vi "Main.vi"(11 "Module Admin":refnum<class "Delacor_lib_QMH_Module Admin.lvclass">) -> ()   [LabVIEW 2020, in "Settings Editor.lvlib"]
doc: "This template is based off of the Queued Message Handler design pattern and the Queued Message Handler project template that ships with LabVIEW.\n\nThe main difference is that the queue is private to this module and communication between modules is performed via Broadcast and Request events.\n\nRequest events are wrapped in public API methods and are handled in the Event Handling Loop (EHL) of this VI. Any module can register for Broadcast events sent by this module. The EHL generates messages based on user interface actions.\n\nThe Message Handling Loop (MHL) processes messages generated by the EHL, or by other messages. The messages are string values, so new messages can be added easily to the Message Cases case structure in the MHL. Each message cluster can also provide an optional value for Message Data, which is a variant that can be converted to whatever message-specific data is required.\n_____\nBased on Delacor QMH Project Template 4.0.0.47.\n_____\nBased on DQMH Project Template 6.0.0.91."
uses:
  Settings Editor.lvlib
  DAQmx Trigger Settings--cluster.ctl
  DAQmx Timing--cluster.ctl
  DAQmx Config--cluster.ctl
  <vilib>/Delacor/Delacor QMH/Libraries/Module Admin_class/Delacor_lib_QMH_Module Admin.lvclass
  Module Data--cluster.ctl
  Settings--cluster.ctl
  Stop Argument--cluster.ctl
  <vilib>/Delacor/Delacor QMH/Libraries/Message Queue_class/Delacor_lib_QMH_Message Queue.lvclass/Delacor_lib_QMH_Message Queue.ctl
  Update Application Settings Argument--cluster.ctl
  Update Application Settings (Reply Payload)--cluster.ctl
  <vilib>/Delacor/Delacor QMH/Libraries/Module Admin_class/Delacor_lib_QMH_Module Admin.lvclass/Delacor_lib_QMH_Module Admin.ctl
  <vilib>/Delacor/Delacor QMH/Libraries/Message Queue_class/Delacor_lib_QMH_Enqueue Message (Single).vi
  <vilib>/Delacor/Delacor QMH/Libraries/Module Admin_class/Delacor_lib_QMH_Get External Launch.vi
  <vilib>/Utility/error.llb/Error Cluster From Error Code.vi
  <vilib>/ErrorRing/Error Ring.xnode
  <vilib>/Delacor/Delacor QMH/Libraries/Message Queue_class/Delacor_lib_QMH_Message Queue.lvclass
panel:
  in  "Config Something":bool
  in  "Config CAM":bool
  in  "Config DAQ":bool
  in  "DAQmx Settings":T1(tab)=enum."Timing Settings"
  in  "Hardware \nConfig Cluster":T2=[{"Physical channels"="Dev1/ai0", "Channel Name"="pd", "Unit"=0, "Min Voltage"=-1.0, "Max Voltage"=1.0}, {"Physical channels"="Dev1/ai1", "Channel Name"="pdh", "Unit"=0, "Min Voltage"=-0.5, "Max Voltage"=0.5}] {"Unit" items=["Volts", "From Custom Scale"]}
  in  "DAQmx \nTiming Settings":T3={"rate"=1000000.0, "source"="OnboardClock", "sample mode"=10178, "samples per channel"=200000} {"sample mode" items=["Finite Samples"=10178, "Continuous Samples"=10123, "Hardware Timed Single Point"=12522]; "rate" format="%0.2f"}
  in  "Trigger Settings":T4={"Trigger Type"=enum."No Trigger", "Digital Start"={"Source"="", "Digital Start Trigger Edge"=10280}, "Digital Pause"={"Source"="", "Digital Pause Trigger Pause When"=10192}, "Digital Reference"={"Source"="", "Digital Start Trigger Edge"=10280, "Digital Reference Pretrigger Samples"=0}, "Analog Start"={"Source"="", "Analog Slope"=10280, "Analog Start Trigger Hysteresis"=0.0, "Analog Start Trigger Level"=0.0}, "Analog Pause"={"Source"="", "Analog Start Trigger Level"=0.0, "Analog Pause Trigger Pause When"=10093}, "Analog Reference"={"Source"="", "Slope"=10280, "Pretrigger Samples"=0, "Level"=0.0}, "Time Start"={"Select Time\nManually"=FALSE, "When"=timestamp(0 s since 1904-01-01)}} {"Time Start"."When" format="%<%x %.3X>T"; "Analog Reference"."Level" format="%0.2f"; "Analog Reference"."Slope" items=["Rising"=10280, "Falling"=10171]; "Analog Pause"."Analog Pause Trigger Pause When" items=["Above Level"=10093, "Below Level"=10107]; "Analog Pause"."Analog Start Trigger Level" format="%0.2f"; "Analog Start"."Analog Start Trigger Level" format="%0.2f"; "Analog Start"."Analog Start Trigger Hysteresis" format="%.2f"; "Analog Start"."Analog Slope" items=["Rising"=10280, "Falling"=10171]; "Digital Reference"."Digital Start Trigger Edge" items=["Rising"=10280, "Falling"=10171]; "Digital Pause"."Digital Pause Trigger Pause When" items=["High"=10192, "Low"=10214]; "Digital Start"."Digital Start Trigger Edge" items=["Rising"=10280, "Falling"=10171]}
  in  "Calibration Array":cluster{"Slope":dbl, "Intercept":dbl}[](array[cluster])=[{"Slope"=1.0, "Intercept"=0.0}, {"Slope"=1.0, "Intercept"=0.0}]
  in  "Cancel":bool
  in  "OK":bool
  in  "Log File Base Path":path=path "C:/Logged Files/26Jan2022/test.tdms"
  out "error out":errorcluster
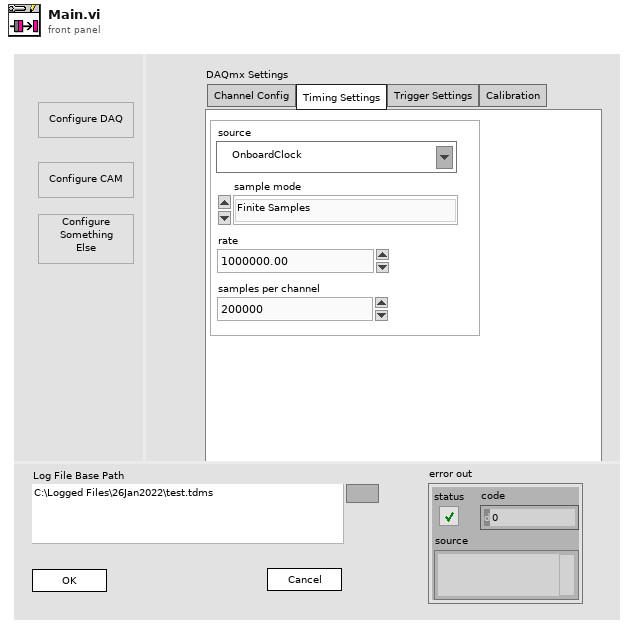
[diagram p1: front panel]
types:
  T1 = enum32{"Channel Config", "Timing Settings", "Trigger Settings", "Calibration"}
  T2 = typedef "Settings Editor.lvlib/DAQmx Config--cluster.ctl" = cluster{"Physical channels":tag, "Channel Name":string, "Unit":i32, "Min Voltage":dbl, "Max Voltage":dbl}[]
  T3 = typedef "Settings Editor.lvlib/DAQmx Timing--cluster.ctl" = cluster{"rate":dbl, "source":tag, "sample mode":i32, "samples per channel":i32}
  T4 = typedef "Settings Editor.lvlib/DAQmx Trigger Settings--cluster.ctl" = cluster{"Trigger Type":enum32{"No Trigger", "Digital Start", "Digital Pause", "Digital Reference", "Analog Start", "Analog Pause", "Analog Reference", "Time Start"}, "Digital Start":cluster{"Source":tag, "Digital Start Trigger Edge":i32}, "Digital Pause":cluster{"Source":tag, "Digital Pause Trigger Pause When":i32}, "Digital Reference":cluster{"Source":tag, "Digital Start Trigger Edge":i32, "Digital Reference Pretrigger Samples":u32}, "Analog Start":cluster{"Source":string, "Analog Slope":i32, "Analog Start Trigger Hysteresis":dbl, "Analog Start Trigger Level":dbl}, "Analog Pause":cluster{"Source":string, "Analog Start Trigger Level":dbl, "Analog Pause Trigger Pause When":i32}, "Analog Reference":cluster{"Source":string, "Slope":i32, "Pretrigger Samples":u32, "Level":dbl}, "Time Start":cluster{"Select Time\nManually":bool, "When":timestamp}}
  T5 = typedef "Settings Editor.lvlib/Request Events--cluster.ctl" = cluster{"Stop Module":refnum<user-event>, "Show Panel":refnum<user-event>, "Hide Panel":refnum<user-event>, "Get Module Execution Status":refnum<user-event>, "Show Diagram":refnum<user-event>, "Update Application Settings":refnum<user-event>}
  T6 = typedef "Settings Editor.lvlib/Module Data--cluster.ctl" = cluster{"Settings":T7}
  T7 = typedef "Settings Editor.lvlib/Settings--cluster.ctl" = cluster{"Calibration Array":cluster{"Slope":dbl, "Offset":dbl}[], "Hardware Config Cluster":T2, "Trigger Settings":T4, "Log File Base Path":path, "DAQmx Timing Settings":T3}
  T8 = enum32{"invalid lock state", "Not Locked", "Locked (No Password)", "Password-protected"}
  T9 = typedef "Settings Editor.lvlib/Stop Argument--cluster.ctl" = cluster{"Origin":string, "Exit via Stop Module Req?":bool, "Wait for Module to stop?":bool}
  T10 = typedef "Settings Editor.lvlib/Update Application Settings Argument--cluster.ctl" = cluster{"Wait Notifier":refnum<notifier>, "wait for reply":bool}
  T11 = enum32{"Invalid", "Standard", "Closed", "Hidden", "Minimized", "Maximized"}
  T12 = typedef "Settings Editor.lvlib/Update Application Settings (Reply Payload)--cluster.ctl" = cluster{"Settings":T7, "Update Settings_error":errorcluster}
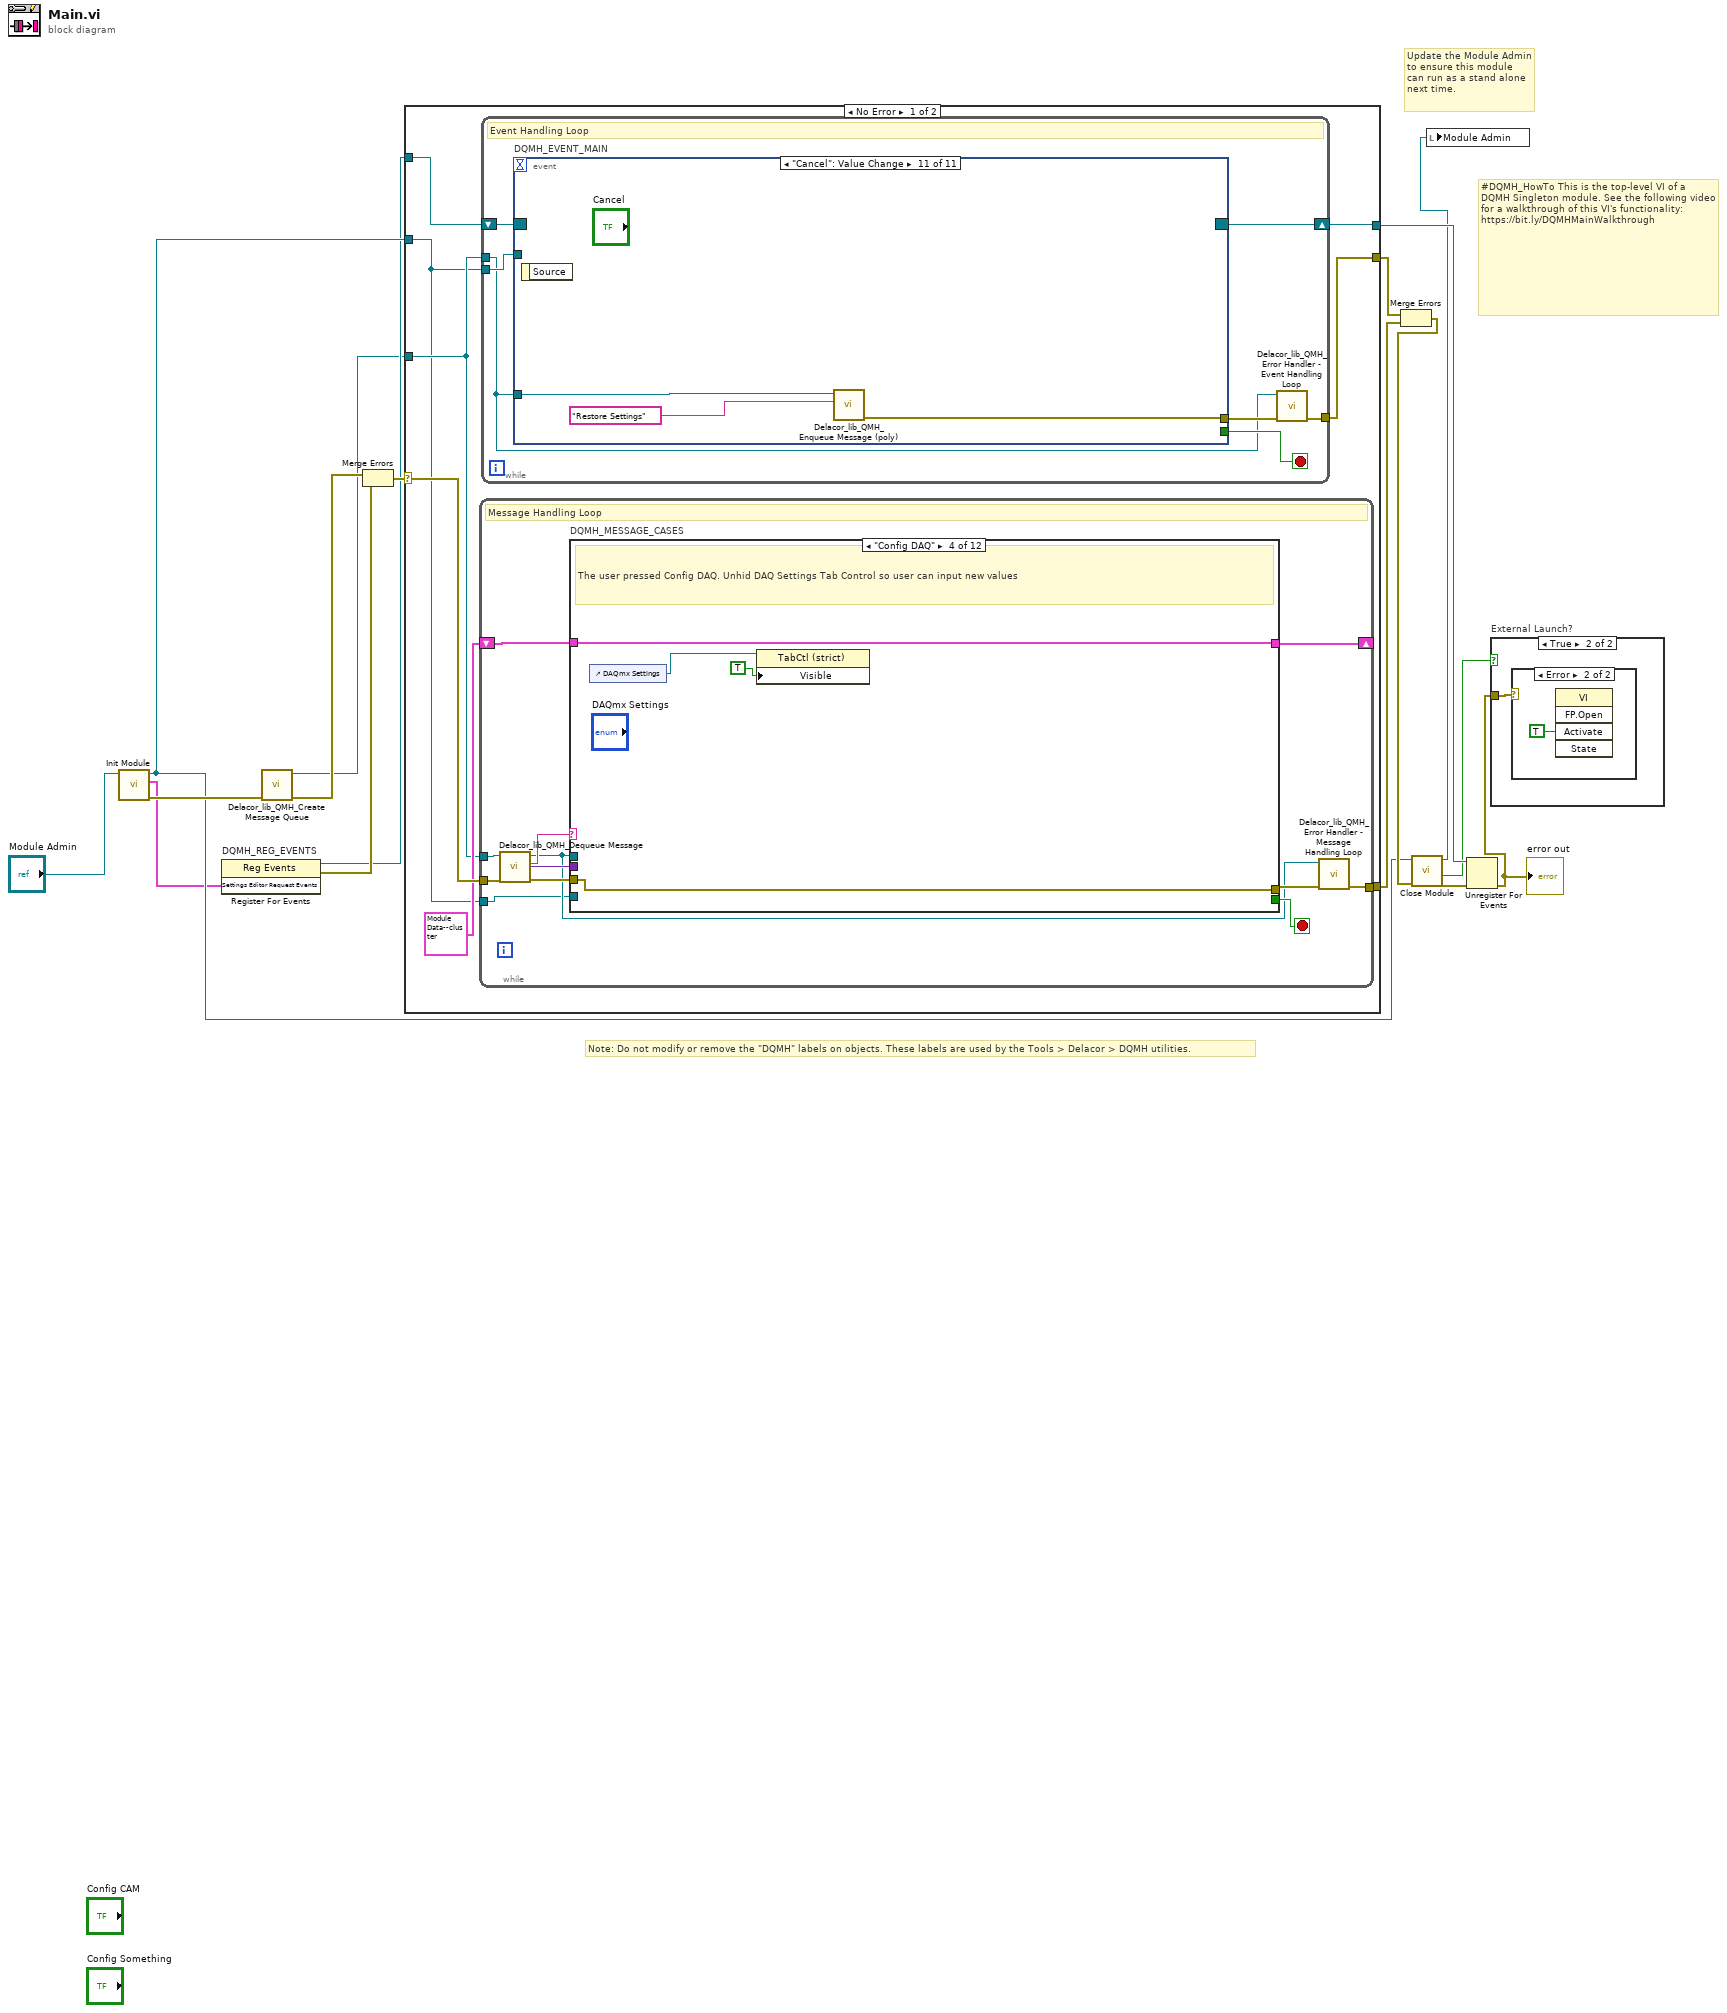
[diagram p0: block diagram]
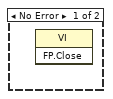
[diagram p3: hidden frame]
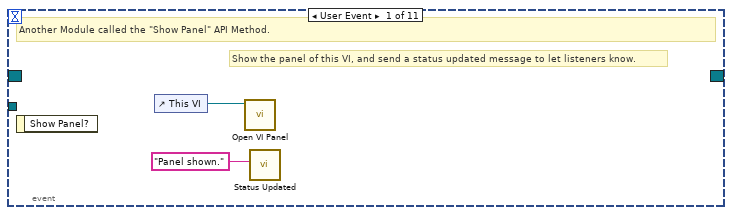
[diagram p4: hidden frame]
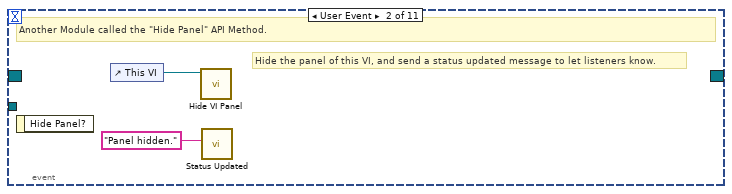
[diagram p5: hidden frame]
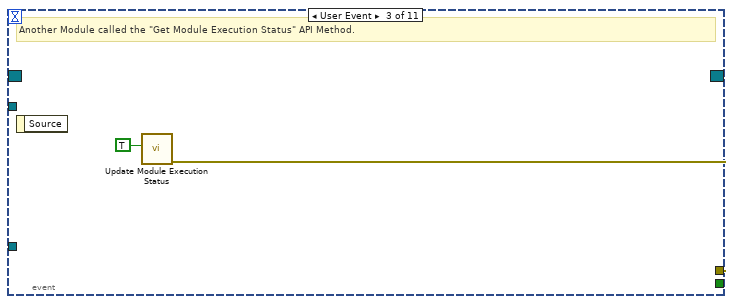
[diagram p6: hidden frame]
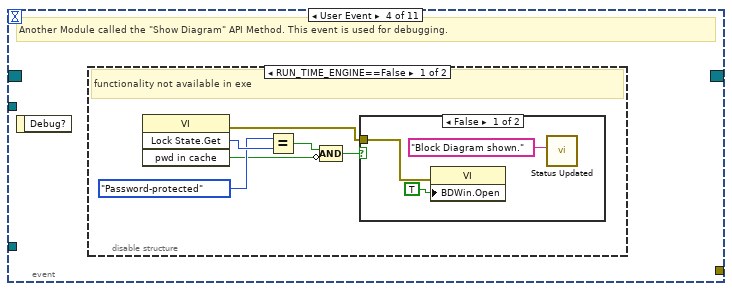
[diagram p7: hidden frame]
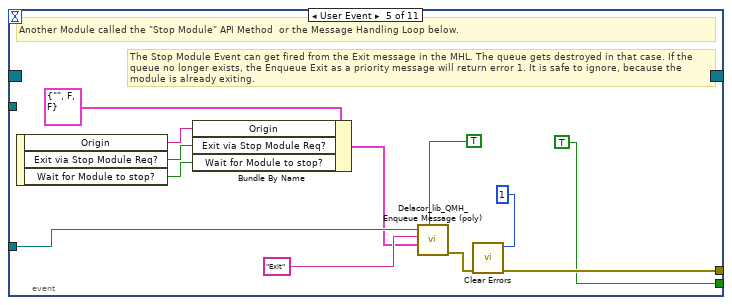
[diagram p10: hidden frame]
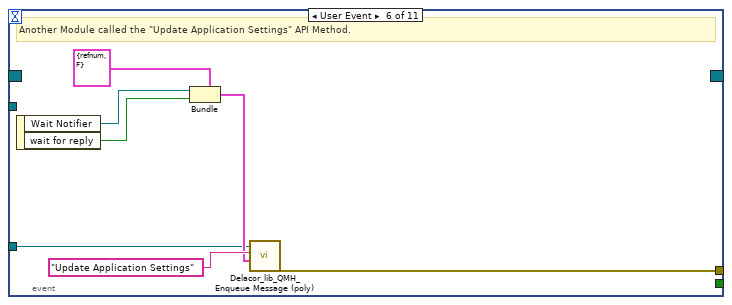
[diagram p11: hidden frame]
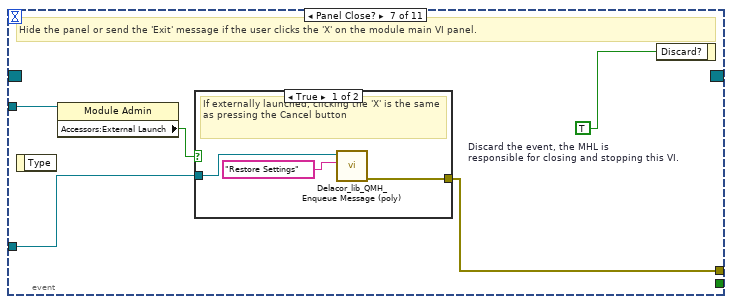
[diagram p12: hidden frame]
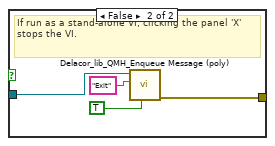
[diagram p13: hidden frame]
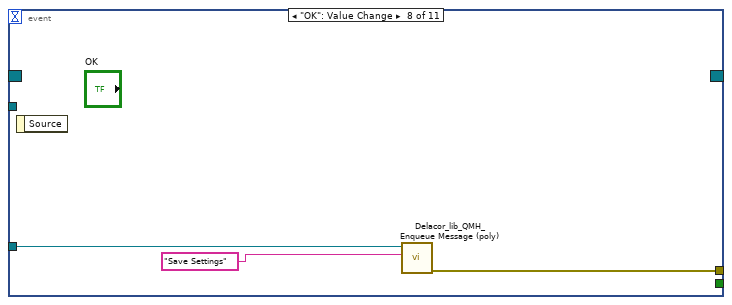
[diagram p14: hidden frame]
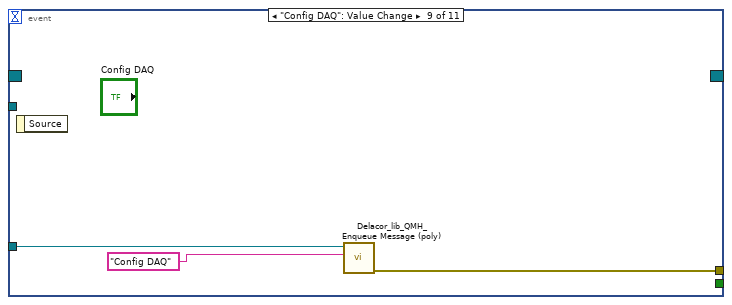
[diagram p15: hidden frame]
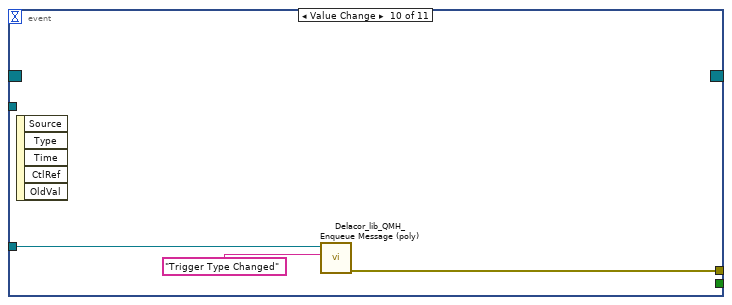
[diagram p16: hidden frame]
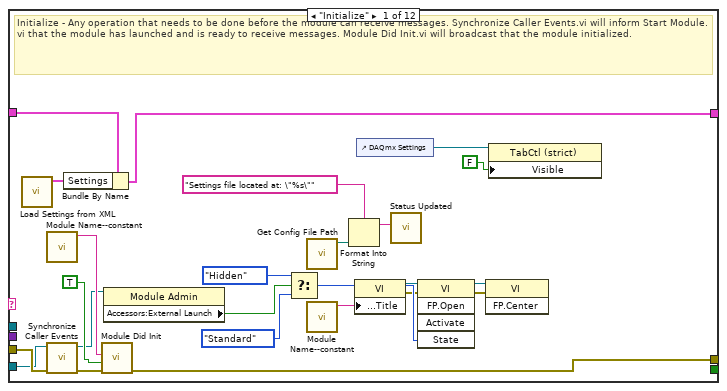
[diagram p17: hidden frame]
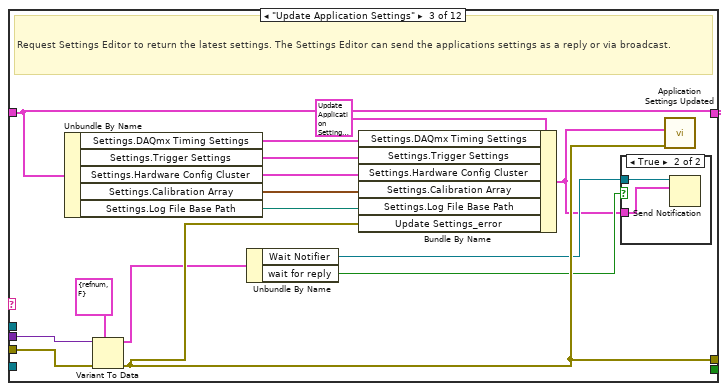
[diagram p19: hidden frame]
diagram:
  # "#DQMH_HowTo This is the top-level VI of a DQMH Singleton module. See the following video for a walkthrough of this VI's functionality: https://bit.ly/DQMHMainWalkthrough"
  # "Note: Do not modify or remove the \"DQMH\" labels on objects. These labels are used by the Tools > Delacor > DQMH utilities."
  # "Update the Module Admin to ensure this module can run as a stand alone next time."
  n1 = call "Init Module.vi"("Singleton Module Admin in"="Module Admin") -> ("error out"=w16:errorcluster, "Settings Editor Request Events"=w5:T5, "Singleton Module Admin out"=w8:refnum<class "Delacor_lib_QMH_Module Admin.lvclass">)  [unwired: 8 in]
  n2 = register-events "DQMH_REG_EVENTS"(w5) -> (reference out=w6:refnum<event-registration>, error out=w9:errorcluster)  [unwired: 2 in]
  n3 = call <vilib>:"Delacor_lib_QMH_Create Message Queue.vi"("error in"=w16) -> ("error out"=w11:errorcluster, "Message Queue"=w4:refnum<class "Delacor_lib_QMH_Message Queue.lvclass">)  [unwired: 9 in]
  n4 = Merge Errors(w11, w9) -> (w10:errorcluster)
  n5 = case shown="No Error" w10 {
    selector: w10 -> [w23 w228]
    tunnel: [w25 w227] -> w17
    tunnel: [w22 w234] -> w7
    tunnel: w6 -> [w20 w234]
    tunnel: w4 -> [w19 w229]
    tunnel: [w24 _] -> w14
    tunnel: w8 -> [w18 w230]
    frame No Error {
      n6 = while {
        tunnel: w19 -> [w93]
        shift-right: [w97] -> _
        shift-left: T6 {"Settings"={"Calibration Array"=[{"Slope"=1.0, "Offset"=0.0}], "Hardware Config Cluster"=[], "Trigger Settings"={"Trigger Type"=enum."No Trigger", "Digital Start"={"Source"="", "Digital Start Trigger Edge"=0}, "Digital Pause"={"Source"="APFI0", "Digital Pause Trigger Pause When"=10192}, "Digital Reference"={"Source"="", "Digital Start Trigger Edge"=10280, "Digital Reference Pretrigger Samples"=0}, "Analog Start"={"Source"="", "Analog Slope"=10093, "Analog Start Trigger Hysteresis"=0.0, "Analog Start Trigger Level"=0.0}, "Analog Pause"={"Source"="", "Analog Start Trigger Level"=0.0, "Analog Pause Trigger Pause When"=10093}, "Analog Reference"={"Source"="", "Slope"=10280, "Pretrigger Samples"=0, "Level"=0.0}, "Time Start"={"Select Time\nManually"=FALSE, "When"=timestamp(0 s since 1904-01-01)}}, "Log File Base Path"=path "", "DAQmx Timing Settings"={"rate"=0.0, "source"="", "sample mode"=0, "samples per channel"=0}}} ("Data Cluster") -> [w98]
        tunnel: w23 -> [w101]
        tunnel: [w99] -> w25
        tunnel: w18 -> [w91]
        stop <- w96 stop-if-true
        # "Message Handling Loop"
        n7 = call-dynamic "Delacor_lib_QMH_Dequeue Message.vi"("error in"=w101, "Message Queue in"=w93) -> ("error out"=w100:errorcluster, "Message Data"=w94:variant, "Message"=w95:string, "Message Queue out"=w92:refnum<class "Delacor_lib_QMH_Message Queue.lvclass">)  [unwired: 6 in]
        n8 = case "DQMH_MESSAGE_CASES" shown="\"Config DAQ\"" w95 {
          selector: w95 -> [_ _ _ _ _ _ _ _ _ _ _ w214]
          tunnel: w92 -> [_ _ _ _ _ _ _ _ _ w184 w206 _]
          tunnel: w100 -> [w125 w128 w142 w149 w151 w165 w171 w179 w181 w191 w212 w216]
          tunnel: [w105 w128 w143 w149 w150 w166 w171 w178 w181 w187 w209 w217] -> w102
          tunnel: w98 -> [w115 w127 w136 w148 w153 w157 w176 w177 w180 w186 w205 w215]
          tunnel: [w114 w127 w136 w148 w153 w154 w176 w177 w180 w186 w205 w215] -> w97
          tunnel: [_ _ _ _ _ _ _ _ _ _ w204 _] -> w96
          tunnel: w94 -> [_ _ w141 _ _ _ _ _ _ w185 w203 _]
          tunnel: w91 -> [w116 _ _ _ _ _ _ _ _ w183 w198 _]
          frame "Initialize" {
            # "Initialize - Any operation that needs to be done before the module can receive messages. Synchronize Caller Events.vi will inform Start Module.vi that the module has launched and is ready to receive messages. Module Did Init.vi will broadcast that the module initialized."
            n9 = call "Load Settings from XML.vi"() -> ("Settings out"=w106:T7)  [unwired: 10 in, 1 out]
            n10 = call "Module Name--constant.vi"() -> ("Module Name"=w112:string)  [unwired: 11 in]
            n11 = call "Synchronize Caller Events.vi"("error in (no error)"=w125, "Singleton Module Admin in"=w116) -> ("error out"=w124:errorcluster, "Singleton Module Admin out"=w111:refnum<class "Delacor_lib_QMH_Module Admin.lvclass">)  [unwired: 8 in]
            n12 = Bundle By Name(cluster=w115, "Settings"=w106) -> (w114:T6)
            n13 = call "Module Did Init.vi"("error in (no error)"=w124, "Initialized?"=TRUE, "Origin"=w112) -> ("error out"=w105:errorcluster)  [unwired: 8 in]
            n14 = property class="Module Admin"(reference=w111) -> ("Accessors:External Launch"=w120:bool)  [unwired: 1 in, 2 out]
            n15 = Select(t=T11."Hidden" ("State"), s=w120, f=T11."Standard" ("State")) -> (s? t:f=w117:T11)
            n16 = call "Get Config File Path.vi"() -> ("XML File Path"=w109:path)  [unwired: 10 in, 1 out]
            n17 = call "Module Name--constant.vi"() -> ("Module Name"=w123:string)  [unwired: 11 in]
            n18 = Format Into String(format string="Settings file located at: \"%s\"", w109) -> (resulting string=w108:string)  [unwired: 2 in, 1 out]
            n19 = property class="VI"("Front Panel.Title"=w123) -> (reference out=w122:refnum<vi>, error out=w110:errorcluster)  [unwired: 2 in]
            n20 = control-ref of="DAQmx Settings"() -> (w104:refnum<vi>)
            n21 = call "Status Updated.vi"("Status"=w108) -> ()  [unwired: 10 in, 1 out]
            n22 = invoke class="VI" method="FP.Open"(reference=w122, error in=w110, "State"=w117) -> (reference out=w121:refnum<vi>, error out=w126:errorcluster)  [unwired: 2 in, 3 out]
            n23 = invoke class="VI" method="FP.Center"(reference=w121, error in=w126) -> ()  [unwired: 1 in, 3 out]
            n24 = property class="TabCtl (strict)"(reference=w104, "Visible"=FALSE) -> ()  [unwired: 1 in, 2 out]
          }
          frame "---Module Specific---" {
            # "Separator -- The following cases handle messages specific to this Module."
          }
          frame "Update Application Settings" {
            # "Request Settings Editor to return the latest settings. The Settings Editor can send the applications settings as a reply or via broadcast."
            n25 = Unbundle By Name(w136) -> ("Settings.DAQmx Timing Settings"=w129:T3, "Settings.Trigger Settings"=w130:T4, "Settings.Hardware Config Cluster"=w131:T2, "Settings.Calibration Array"=w134:cluster{"Slope":dbl, "Offset":dbl}[], "Settings.Log File Base Path"=w133:path)
            n26 = Variant To Data(error in=w142, type=T10 {"Wait Notifier"=refnum, "wait for reply"=FALSE} ("Update Application Settings Argument"), Variant=w141) -> (data=w139:T10, error out=w143:errorcluster)
            n27 = Unbundle By Name(w139) -> ("Wait Notifier"=w138:refnum<notifier>, "wait for reply"=w137:bool)
            n28 = Bundle By Name(cluster=T12 {"Settings"={"Calibration Array"=[], "Hardware Config Cluster"=[], "Trigger Settings"={"Trigger Type"=enum."No Trigger", "Digital Start"={"Source"="", "Digital Start Trigger Edge"=0}, "Digital Pause"={"Source"="APFI0", "Digital Pause Trigger Pause When"=10192}, "Digital Reference"={"Source"="", "Digital Start Trigger Edge"=10280, "Digital Reference Pretrigger Samples"=0}, "Analog Start"={"Source"="", "Analog Slope"=10093, "Analog Start Trigger Hysteresis"=0.0, "Analog Start Trigger Level"=0.0}, "Analog Pause"={"Source"="", "Analog Start Trigger Level"=0.0, "Analog Pause Trigger Pause When"=10093}, "Analog Reference"={"Source"="", "Slope"=10280, "Pretrigger Samples"=0, "Level"=0.0}, "Time Start"={"Select Time\nManually"=FALSE, "When"=timestamp(0 s since 1904-01-01)}}, "Log File Base Path"=path "", "DAQmx Timing Settings"={"rate"=0.0, "source"="", "sample mode"=0, "samples per channel"=0}}, "Update Settings_error"={"status"=FALSE, "code"=0, "source"=""}} ("Update Application Settings (Reply Payload)"), "Settings.DAQmx Timing Settings"=w129, "Settings.Trigger Settings"=w130, "Settings.Hardware Config Cluster"=w131, "Settings.Calibration Array"=w134, "Settings.Log File Base Path"=w133, "Update Settings_error"=w143) -> (w132:T12)
            n29 = case shown="True" w137 {
              tunnel: w138 -> [_ w145]
              tunnel: w132 -> [_ w144]
              frame False {
              }
              frame True {
                n30 = Send Notification(notification=w144, notifier=w145) -> ()  [unwired: 1 in, 2 out]
              }
            }
            n31 = call "Application Settings Updated.vi"("error in (no error)"=w143, "Reply Payload"=w132) -> ()  [unwired: 9 in, 1 out]
          }
          frame "Config DAQ" {
            # "The user pressed Config DAQ. Unhid DAQ Settings Tab Control so user can input new values"
            n32 = control-ref of="DAQmx Settings"() -> (w146:refnum<vi>)
            n33 = property class="TabCtl (strict)"(reference=w146, "Visible"=TRUE) -> ()  [unwired: 1 in, 2 out]
          }
          frame "Trigger Type Changed" {
            # "User changed the trigger type. Unhide the options of the new trigger type."
            n34 = control-ref of="Trigger Settings"() -> (w152:refnum<vi>)
            n35 = call "Trigger Selection Display.vi"("error in (no error)"=w151, "reference"=w152) -> ("error out"=w150:errorcluster)  [unwired: 9 in]
          }
          frame "Save Settings" {
            # "The end user pressed OK button and the current values on the front panel are the new settings."
            n36 = Bundle By Name(cluster=w157, "Settings.Hardware Config Cluster"="Hardware \nConfig Cluster", "Settings.DAQmx Timing Settings"="DAQmx \nTiming Settings", "Settings.Trigger Settings"="Trigger Settings", "Settings.Calibration Array"="Calibration Array", "Settings.Log File Base Path"="Log File Base Path") -> (w154:T6)
            n37 = Unbundle By Name(w154) -> ("Settings"=w155:T7)
            n38 = Bundle By Name(cluster=T12 {"Settings"={"Calibration Array"=[], "Hardware Config Cluster"=[], "Trigger Settings"={"Trigger Type"=enum."No Trigger", "Digital Start"={"Source"="", "Digital Start Trigger Edge"=0}, "Digital Pause"={"Source"="APFI0", "Digital Pause Trigger Pause When"=10192}, "Digital Reference"={"Source"="", "Digital Start Trigger Edge"=10280, "Digital Reference Pretrigger Samples"=0}, "Analog Start"={"Source"="", "Analog Slope"=10093, "Analog Start Trigger Hysteresis"=0.0, "Analog Start Trigger Level"=0.0}, "Analog Pause"={"Source"="", "Analog Start Trigger Level"=0.0, "Analog Pause Trigger Pause When"=10093}, "Analog Reference"={"Source"="", "Slope"=10280, "Pretrigger Samples"=0, "Level"=0.0}, "Time Start"={"Select Time\nManually"=FALSE, "When"=timestamp(0 s since 1904-01-01)}}, "Log File Base Path"=path "", "DAQmx Timing Settings"={"rate"=0.0, "source"="", "sample mode"=0, "samples per channel"=0}}, "Update Settings_error"={"status"=FALSE, "code"=0, "source"=""}} ("Reply Payload"), "Settings"=w155) -> (w156:T12)
            n39 = control-ref of="This VI"() -> (w168:refnum<vi>)
            n40 = call "Hide VI Panel.vi"("VI"=w168) -> ()  [unwired: 10 in, 1 out]
            n41 = call "Application Settings Updated.vi"("Reply Payload"=w156) -> ("error out"=w163:errorcluster)  [unwired: 10 in]
            n42 = call "Save Settings to XML.vi"("Settings"=w155) -> ("error out"=w164:errorcluster)  [unwired: 10 in]
            n43 = Merge Errors(w165, w164, w163) -> (w166:errorcluster)
          }
          frame "Restore Settings" {
            # "The end user pressed Cancel button, need to restore the current stored values for the controls on the front panel. No need to broadcast that the settings changed."
            n44 = Unbundle By Name(w176) -> ("Settings.Calibration Array"=w174:cluster{"Slope":dbl, "Offset":dbl}[], "Settings.Log File Base Path"=w173:path, "Settings.DAQmx Timing Settings"=w172:T3, "Settings.Trigger Settings"=w170:T4, "Settings.Hardware Config Cluster"=w169:T2)
            n45 = control-ref of="This VI"() -> (w175:refnum<vi>)
            n46 = call "Hide VI Panel.vi"("VI"=w175) -> ()  [unwired: 10 in, 1 out]
            n47 = local write "Hardware \nConfig Cluster"(w169) -> ()
            n48 = local write "DAQmx \nTiming Settings"(w172) -> ()
            n49 = local write "Log File Base Path"(w173) -> ()
            n50 = local write "Calibration Array"(w174) -> ()
            n51 = local write "Trigger Settings"(w170) -> ()
          }
          frame "---Copy This Frame---" {
            # "Duplicate this frame when creating new messages.  Change this comment in the duplicated frame to describe this message."
            n52 = Merge Errors(w179) -> (w178:errorcluster)
          }
          frame "---Exit and Error Handling---" {
            # "Separator - The following cases handle errors and exit messages."
          }
          frame "Error" {
            # "Error - Check the error message data and respond accordingly. This message is sent by the \"Error Handler\" VIs at the end of each loop in this application."
            n53 = property class="Module Admin"(reference=w183) -> ("Accessors:External Launch"=w182:bool)  [unwired: 1 in, 2 out]
            n54 = Variant To Data(error in=w191, type=errorcluster {"status"=FALSE, "code"=0, "source"=""} ("error constant"), Variant=w185) -> (data=w192:errorcluster, error out=w189:errorcluster)
            n55 = case shown="False" w182 {
              tunnel: [w197 _] -> w188
              tunnel: w184 -> [w195 _]
              tunnel: w192 -> [w196 _]
              frame False {
                # "If the module is running standalone, then pop up an error dialog and call the \"Exit\" message."
                n56 = call <vilib>:"Simple Error Handler.vi"("error in (no error)"=w196) -> ()  [unwired: 4 in, 5 out]
                n57 = call-poly <vilib>:"Delacor_lib_QMH_Enqueue Message (poly).vi"("Priority Message? (F)"=TRUE, "Message"="Exit", "Message Queue in"=w195) -> ("error out"=w197:errorcluster)  [unwired: 7 in, 1 out]
              }
              frame True {
                # "If the module was launched externally, calling the Error Reported broadcast VI is the only action performed by the \"Error\" message. The module's caller can then process the error appropriately."
              }
            }
            n58 = call "Error Reported.vi"("Error"=w192) -> ()  [unwired: 10 in, 1 out]
            n59 = Merge Errors(w189, w188) -> (w187:errorcluster)
            n60 = local write "error out"(w187) -> ()
          }
          frame "Exit" {
            w202 = 91  # 91: not all Exit messages will have an argument
            w204 = TRUE  # Stop the VI
            # "Release the message queue reference"
            # "Exit - Exit the application."
            n61 = Variant To Data(error in=w212, type=T9 {"Origin"="", "Exit via Stop Module Req?"=FALSE, "Wait for Module to stop?"=FALSE} ("Stop Argument"), Variant=w203) -> (data=w200:T9, error out=w208:errorcluster)
            n62 = call <vilib>:"Clear Errors.vi"("error in (no error)"=w208, "specific error code to clear (0: all)"=w202) -> ("error out"=w211:errorcluster)  [unwired: 4 in, 1 out]
            n63 = control-ref of="This VI"() -> (w199:refnum<vi>)
            n64 = call "Handle Exit.vi"("Stop Argument"=w200, "Admin in"=w198, "VI reference"=w199) -> ("error out"=w207:errorcluster)  [unwired: 7 in, 1 out]
            n65 = call-dynamic "Delacor_lib_QMH_Release Message Queue.vi"("error in"=w211, "Message Queue"=w206) -> ("error out"=w210:errorcluster)  [unwired: 9 in]
            n66 = Merge Errors(w210, w207) -> (w209:errorcluster)
          }
          frame Default {
            # "'Default' case only runs if there is a message that isn't defined in any of the other cases.  Output a programming error."
            n67 = call "Module Name--constant.vi"() -> ("Module Name"=w213:string)  [unwired: 11 in]
            n68 = xnode "Error Ring"("parameter 0"=w214, "parameter 1"=w213) -> ("error out"=w218:errorcluster)
            n69 = Merge Errors(w216, w218) -> (w217:errorcluster)
          }
        }
        n70 = call-dynamic "Delacor_lib_QMH_Error Handler - Message Handling Loop.vi"("error in"=w102, "Message Queue in"=w92) -> ("dup error in"=w99:errorcluster)  [unwired: 8 in, 1 out]
      }
      n71 = while {
        tunnel: w19 -> [w26]
        shift-right: [w29] -> w22
        shift-left: w20 -> [w30]
        tunnel: [w31] -> w24
        tunnel: w18 -> [w27]
        stop <- w28 stop-if-true
        # "Event Handling Loop"
        n72 = event "DQMH_EVENT_MAIN" shown="[10] \"Cancel\": Value Change" {
          selector: w30 -> [_ _ _ _ _ _ _ _ _ _ _]
          dyn-events: [_ _ _ _ _ _ _ _ _ _ _] -> w29
          timeout: _ -> [_ _ _ _ _ _ _ _ _ _ _]
          tunnel: [_ _ _ _ TRUE ("Discard?") _ _ _ _ _ _] -> w28
          tunnel: w26 -> [_ _ _ _ w55 w60 w69 w79 w84 w87 w89]
          tunnel: [_ _ w38 _ w58 w63 w71 w80 w83 w86 w88] -> w32
          tunnel: w27 -> [_ _ _ _ _ _ w68 _ _ _ _]
          event User Event {
            # "Show the panel of this VI, and send a status updated message to let listeners know."
            # "Another Module called the \"Show Panel\" API Method."
            n73 = event-data() -> ()  [unwired: 1 in, 1 out]
            n74 = control-ref of="This VI"() -> (w34:refnum<vi>)
            n75 = call "Open VI Panel.vi"("VI"=w34) -> ()  [unwired: 10 in, 1 out]
            n76 = call "Status Updated.vi"("Status"="Panel shown." ("format string")) -> ()  [unwired: 10 in, 1 out]
          }
          event User Event {
            # "Hide the panel of this VI, and send a status updated message to let listeners know."
            # "Another Module called the \"Hide Panel\" API Method."
            n77 = event-data() -> ()  [unwired: 1 in, 1 out]
            n78 = control-ref of="This VI"() -> (w36:refnum<vi>)
            n79 = call "Hide VI Panel.vi"("VI"=w36) -> ()  [unwired: 10 in, 1 out]
            n80 = call "Status Updated.vi"("Status"="Panel hidden." ("format string")) -> ()  [unwired: 10 in, 1 out]
          }
          event User Event {
            # "Another Module called the \"Get Module Execution Status\" API Method."
            n81 = event-data() -> ()  [unwired: 1 in, 1 out]
            n82 = call "Update Module Execution Status.vi"("Running?"=TRUE) -> ("error out"=w38:errorcluster)  [unwired: 10 in]
          }
          event User Event {
            # "Another Module called the \"Show Diagram\" API Method. This event is used for debugging."
            n83 = event-data() -> ()  [unwired: 1 in, 1 out]
            n84 = disable-structure shown="RUN_TIME_ENGINE==False" {
              frame condition #0 (active) {
                # "functionality not available in exe"
                n85 = invoke class="VI" method="Lock State.Get"() -> (error out=w44:errorcluster, "Get Lock State"=w43:T8, "pwd in cache"=w40:bool)  [unwired: 4 in, 1 out]
                n86 = Equal?(x=T8."Password-protected", y=w43) -> (x = y?=w41:bool)
                n87 = Compound Arithmetic op=AND(w41, invert w40) -> (w39:bool)
                n88 = case shown="False" w39 {
                  tunnel: w44 -> [w47 _]
                  frame False {
                    n89 = property class="VI"(error in=w47, "BDWin.Open"=TRUE ("Block Diagram Window:Open")) -> ()  [unwired: 1 in, 2 out]
                    n90 = call "Status Updated.vi"("Status"="Block Diagram shown." ("format string")) -> ()  [unwired: 10 in, 1 out]
                  }
                  frame True {
                    # "Password-protected VI, and the password is not in the cache. Do not show the diagram."
                  }
                }
              }
              frame condition #1 {
              }
            }
          }
          event User Event {
            # "The Stop Module Event can get fired from the Exit message in the MHL. The queue gets destroyed in that case. If the queue no longer exists, the Enqueue Exit as a priority message will return error 1. It is safe to ignore, because the module is already exiting."
            # "Another Module called the \"Stop Module\" API Method  or the Message Handling Loop below."
            n91 = event-data() -> ("Origin"=w48:string, "Exit via Stop Module Req?"=w51:bool, "Wait for Module to stop?"=w50:bool)  [unwired: 1 in]
            n92 = Bundle By Name(cluster=T9 {"Origin"="", "Exit via Stop Module Req?"=FALSE, "Wait for Module to stop?"=FALSE} ("Stop Argument"), "Origin"=w48, "Exit via Stop Module Req?"=w51, "Wait for Module to stop?"=w50) -> (w49:T9)
            n93 = call-poly <vilib>:"Delacor_lib_QMH_Enqueue Message (poly).vi"("Priority Message? (F)"=TRUE, "Message Data"=w49, "Message"="Exit", "Message Queue in"=w55) -> ("error out"=w59:errorcluster)  [unwired: 6 in, 1 out]
            n94 = call <vilib>:"Clear Errors.vi"("error in (no error)"=w59, "specific error code to clear (0: all)"=1) -> ("error out"=w58:errorcluster)  [unwired: 4 in, 1 out]
          }
          event User Event {
            # "Another Module called the \"Update Application Settings\" API Method."
            n95 = event-data() -> ("Wait Notifier"=w62:refnum<notifier>, "wait for reply"=w61:bool)  [unwired: 1 in]
            n96 = Bundle(cluster=T10 {"Wait Notifier"=refnum, "wait for reply"=FALSE} ("Update Application Settings Argument"), "Wait Notifier"=w62, "wait for reply"=w61) -> (w64:T10)
            n97 = call-poly <vilib>:"Delacor_lib_QMH_Enqueue Message (poly).vi"("Message Data"=w64, "Message"="Update Application Settings", "Message Queue in"=w60) -> ("error out"=w63:errorcluster)  [unwired: 7 in, 1 out]
          }
          event Panel Close? {
            w70 = TRUE  # Discard the event, the MHL is  responsible for closing and stopping this VI.
            # "Hide the panel or send the 'Exit' message if the user clicks the 'X' on the module main VI panel."
            n98 = event-data() -> ()  [unwired: 1 in, 1 out]
            n99 = property class="Module Admin"(reference=w68) -> ("Accessors:External Launch"=w67:bool)  [unwired: 1 in, 2 out]
            n100 = case shown="True" w67 {
              tunnel: w69 -> [w73 w77]
              tunnel: [w72 w78] -> w71
              frame True {
                # "If externally launched, clicking the 'X' is the same as pressing the Cancel button"
                n101 = call-poly <vilib>:"Delacor_lib_QMH_Enqueue Message (poly).vi"("Message"="Restore Settings", "Message Queue in"=w73) -> ("error out"=w72:errorcluster)  [unwired: 8 in, 1 out]
              }
              frame False {
                # "If run as a stand-alone VI, clicking the panel 'X' stops the VI."
                n102 = call-poly <vilib>:"Delacor_lib_QMH_Enqueue Message (poly).vi"("Priority Message? (F)"=TRUE, "Message"="Exit", "Message Queue in"=w77) -> ("error out"=w78:errorcluster)  [unwired: 7 in, 1 out]
              }
            }
            n103 = event-data("Discard?"=w70) -> ()  [unwired: 1 in, 1 out]
          }
          event "OK": Value Change {
            n104 = event-data() -> ()  [unwired: 1 in, 1 out]
            n105 = call-poly <vilib>:"Delacor_lib_QMH_Enqueue Message (poly).vi"("Message"="Save Settings", "Message Queue in"=w79) -> ("error out"=w80:errorcluster)  [unwired: 8 in, 1 out]
          }
          event "Config DAQ": Value Change {
            n106 = event-data() -> ()  [unwired: 1 in, 1 out]
            n107 = call-poly <vilib>:"Delacor_lib_QMH_Enqueue Message (poly).vi"("Message"="Config DAQ", "Message Queue in"=w84) -> ("error out"=w83:errorcluster)  [unwired: 8 in, 1 out]
          }
          event Value Change {
            n108 = event-data() -> ()  [unwired: 1 in, 5 out]
            n109 = call-poly <vilib>:"Delacor_lib_QMH_Enqueue Message (poly).vi"("Message"="Trigger Type Changed", "Message Queue in"=w87) -> ("error out"=w86:errorcluster)  [unwired: 8 in, 1 out]
          }
          event "Cancel": Value Change {
            n110 = event-data() -> ()  [unwired: 1 in, 1 out]
            n111 = call-poly <vilib>:"Delacor_lib_QMH_Enqueue Message (poly).vi"("Message"="Restore Settings", "Message Queue in"=w89) -> ("error out"=w88:errorcluster)  [unwired: 8 in, 1 out]
          }
        }
        n112 = call-dynamic "Delacor_lib_QMH_Error Handler - Event Handling Loop.vi"("error in"=w32, "Message Queue in"=w26) -> ("dup error in"=w31:errorcluster)  [unwired: 8 in, 1 out]
      }
    }
    frame Error {
      # "Synchronize Caller Events.vi will inform Start Module.vi that the module has launched and will let the code calling Start Module.vi register for broadcasts and would permit the caller receive the broadcast that an error occurred at launch time."
      n113 = call "Synchronize Caller Events.vi"("Singleton Module Admin in"=w230) -> ("error out"=w235:errorcluster)  [unwired: 9 in, 1 out]
      n114 = call-dynamic "Delacor_lib_QMH_Release Message Queue.vi"("error in"=w228, "Message Queue"=w229) -> ("error out"=w227:errorcluster)  [unwired: 9 in]
      n115 = call "Module Name--constant.vi"() -> ("Module Name"=w233:string)  [unwired: 11 in]
      n116 = Merge Errors(w227, w235) -> (w236:errorcluster)
      n117 = Format Into String(format string="An error occurred during initialization. %s is no longer running.", w233) -> (resulting string=w231:string)  [unwired: 2 in, 1 out]
      n118 = call "Error Reported.vi"("Additional Information"=w231, "Error"=w236) -> ()  [unwired: 9 in, 1 out]
    }
  }
  n119 = Merge Errors(w14, w17) -> (w13:errorcluster)
  n120 = call "Close Module.vi"("error in (no error)"=w13, "Module Admin in"=w8) -> ("error out"=w15:errorcluster, "External Launch"=w1:bool, "Module Admin out"=w2:refnum<class "Delacor_lib_QMH_Module Admin.lvclass">)  [unwired: 7 in]
  n121 = local write "Module Admin"(w2) -> ()
  n122 = Unregister For Events(event registration refnum=w7, error in=w15) -> (error out=w12:errorcluster)
  "error out" <- w12
  n123 = case "External Launch?" shown="True" w1 {
    tunnel: w12 -> [_ w237]
    frame False {
    }
    frame True {
      n124 = case shown="Error" w237 {
        frame No Error {
          n125 = invoke class="VI" method="FP.Close"() -> ()  [unwired: 3 in, 3 out]
        }
        frame Error {
          n126 = invoke class="VI" method="FP.Open"("Activate"=TRUE ("Activate?")) -> ()  [unwired: 4 in, 5 out]
        }
      }
    }
  }
